vi "Get item by index.vi"(8 "error in (no error)":errorcluster caption="错误输入（无错误）", 10 "Index":i32, 11 "Dictionary In":refnum<class "Dictionary.lvclass"> caption="DNL_LabVIEW Object in") -> (0 "error out":errorcluster caption="错误输出", 1 "Value":string, 2 "Key":string, 3 "Dictionary Out":refnum<class "Dictionary.lvclass"> caption="DNL_LabVIEW Object out")   [LabVIEW 2012, in "Dictionary.lvclass"]
uses:
  Dictionary.lvclass
  Dictionary.lvclass/Dictionary.ctl
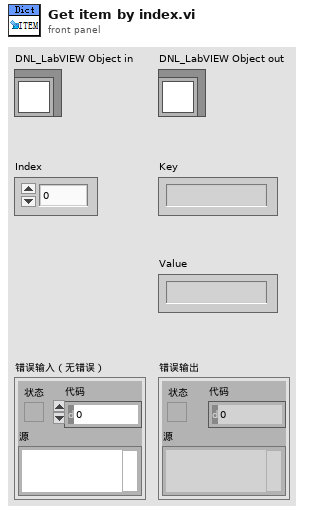
[diagram p1: front panel]
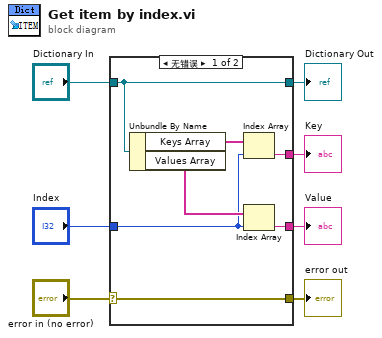
[diagram p0: block diagram]
diagram:
  n1 = case shown="无错误" "error in (no error)" {
    selector: "error in (no error)" -> [w14 w16]
    tunnel: [w14 w16] -> w6
    tunnel: [w13 w15] -> w4
    tunnel: "Dictionary In" -> [w13 w15]
    tunnel: "Index" -> [w10 _]
    tunnel: [w9 _] -> w2
    tunnel: [w8 _] -> w1
    frame No Error {
      n2 = Unbundle By Name(w13) -> ("Keys Array"=w12:string[], "Values Array"=w11:string[])
      n3 = Index Array(array=w12, index=w10) -> (element=w9:string)
      n4 = Index Array(array=w11, index=w10) -> (element=w8:string)
    }
    frame Error {
    }
  }
  "error out" <- w6
  "Dictionary Out" <- w4
  "Key" <- w2
  "Value" <- w1
